vi "mules_modify_caption.vi"(10 "Tip Strip Array":string[](array[string]), 11 "Controls":refnum<vi>[](array[refnum])) -> ()   [LabVIEW 2013]
doc: "Sets all the controls in the input array to the \"Enable state\" value."
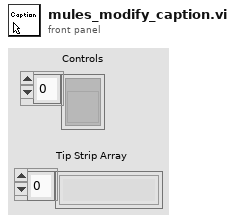
[diagram p1: front panel]
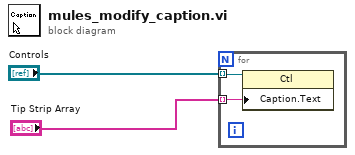
[diagram p0: block diagram]
diagram:
  n1 = for {
    tunnel: "Controls" -> [w4] mode=indexing
    tunnel: "Tip Strip Array" -> [w3] mode=indexing
    n2 = property class="Ctl"(reference=w4, "Caption.Text"=w3) -> ()  [unwired: 1 in, 2 out]
  }
